vi "SetDisplayText.vi"(8 "Error In":errorcluster, 9 "Text (12 Characters)":string, 11 "Keithley 6485 In":refnum<visa-resource-name>) -> (0 "Error Out":errorcluster, 3 "Keithley 6485 Out":refnum<visa-resource-name>)   [LabVIEW 2012, in "Keithley-6485.lvlib"]
uses:
  Keithley-6485.lvlib
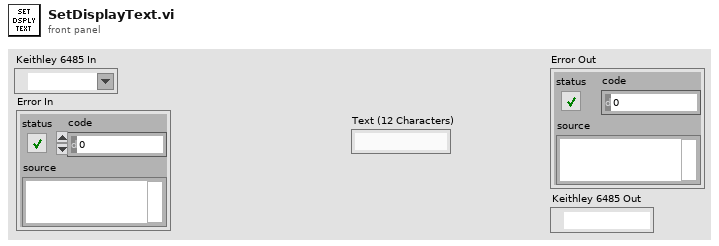
[diagram p1: front panel]
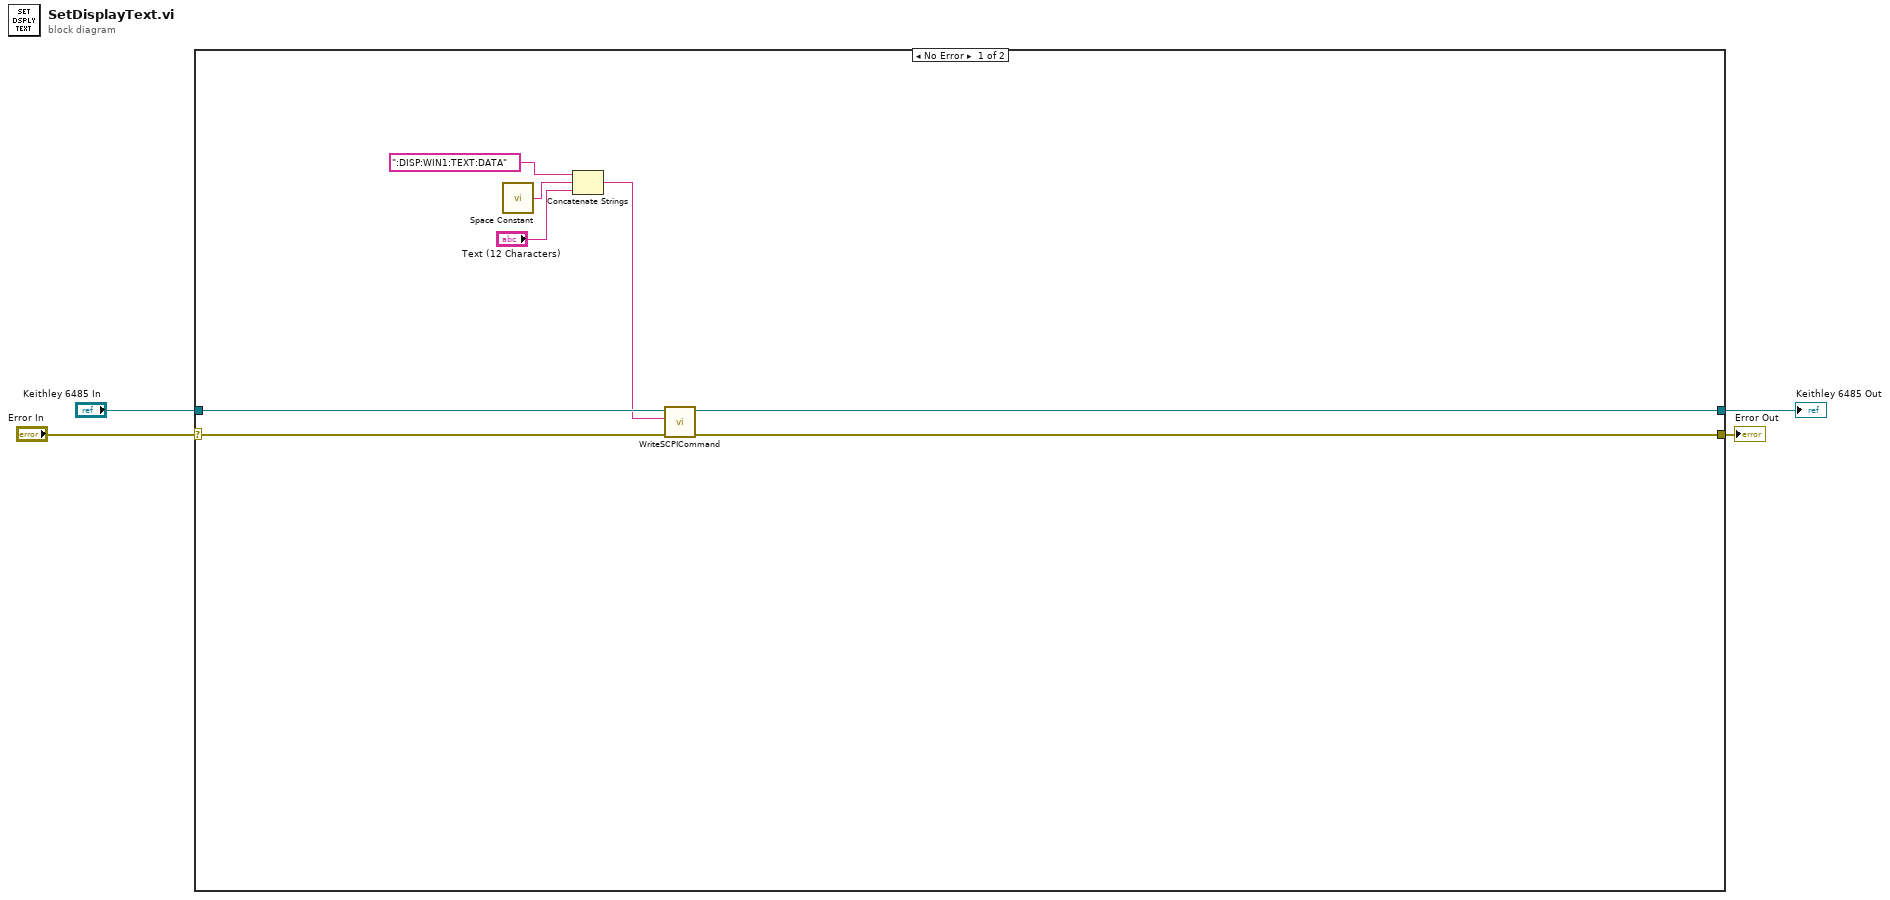
[diagram p0: block diagram]
diagram:
  n1 = case shown="No Error" "Error In" {
    selector: "Error In" -> [w8 w13]
    tunnel: "Keithley 6485 In" -> [w11 w14]
    tunnel: [w9 w13] -> w2
    tunnel: [w10 w14] -> w1
    frame No Error {
      n2 = call <vilib>:"Space Constant.vi"() -> ("String"=w12:string)
      n3 = Concatenate Strings(":DISP:WIN1:TEXT:DATA", w12, "Text (12 Characters)") -> (w7:string)
      n4 = call "WriteSCPICommand.vi"("Error In"=w8, "SCPI Command"=w7, "Keithley 6482 In"=w11) -> ("Error Out"=w9:errorcluster, "Keithley 6482 Out"=w10:refnum<visa-resource-name>)  [unwired: 7 in]
    }
    frame Error {
    }
  }
  "Error Out" <- w2
  "Keithley 6485 Out" <- w1
